vi "NET Control Test.vi"() -> ()   [LabVIEW 2012]
uses:
  NationalInstruments.VeriStand.SystemStorageUI
  NationalInstruments.VeriStand.SystemDefinitionAPI
  NationalInstruments.VeriStand.SystemStorage
  <vilib>/NI VeriStand/UI Controls/Single Node Browser/NI_VS UI Single Node Browser.lvlib
panel:
  out "Numeric":dbl
  in  "Start Trigger Channel":string
  in  "Select Start Trig":bool
  in  "stop":bool
  in  "Path":path=path "C:/Users/Public/Documents/National Instruments/NI VeriStand 2012/Projects/Untitled 1/Untitled 1.nivssdf"
  in  "Source Waveform":refnum<k24>(container)
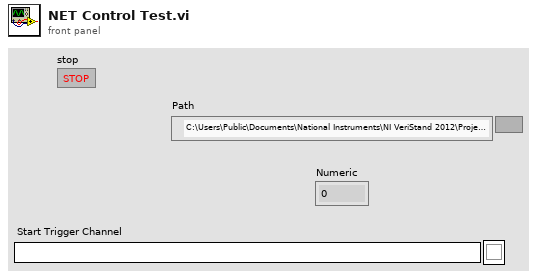
[diagram p1: front panel]
types:
  T1 = typedef "NI_VS UI Single Node Browser.lvlib/Callback Type.ctl" = cluster{"Net Callbacks":refnum<k27>[], "Event":refnum<user-event>}
  T2 = typedef "NI_VS UI Single Node Browser.lvlib/Single Node Browser Ref.ctl" = refnum<k24>
  T3 = typedef "NI_VS UI Single Node Browser.lvlib/Net Event.ctl" = enum16{"SelectedItem"}
  T4 = typedef "NI_VS UI Single Node Browser.lvlib/Node Ref.ctl" = refnum<k24>
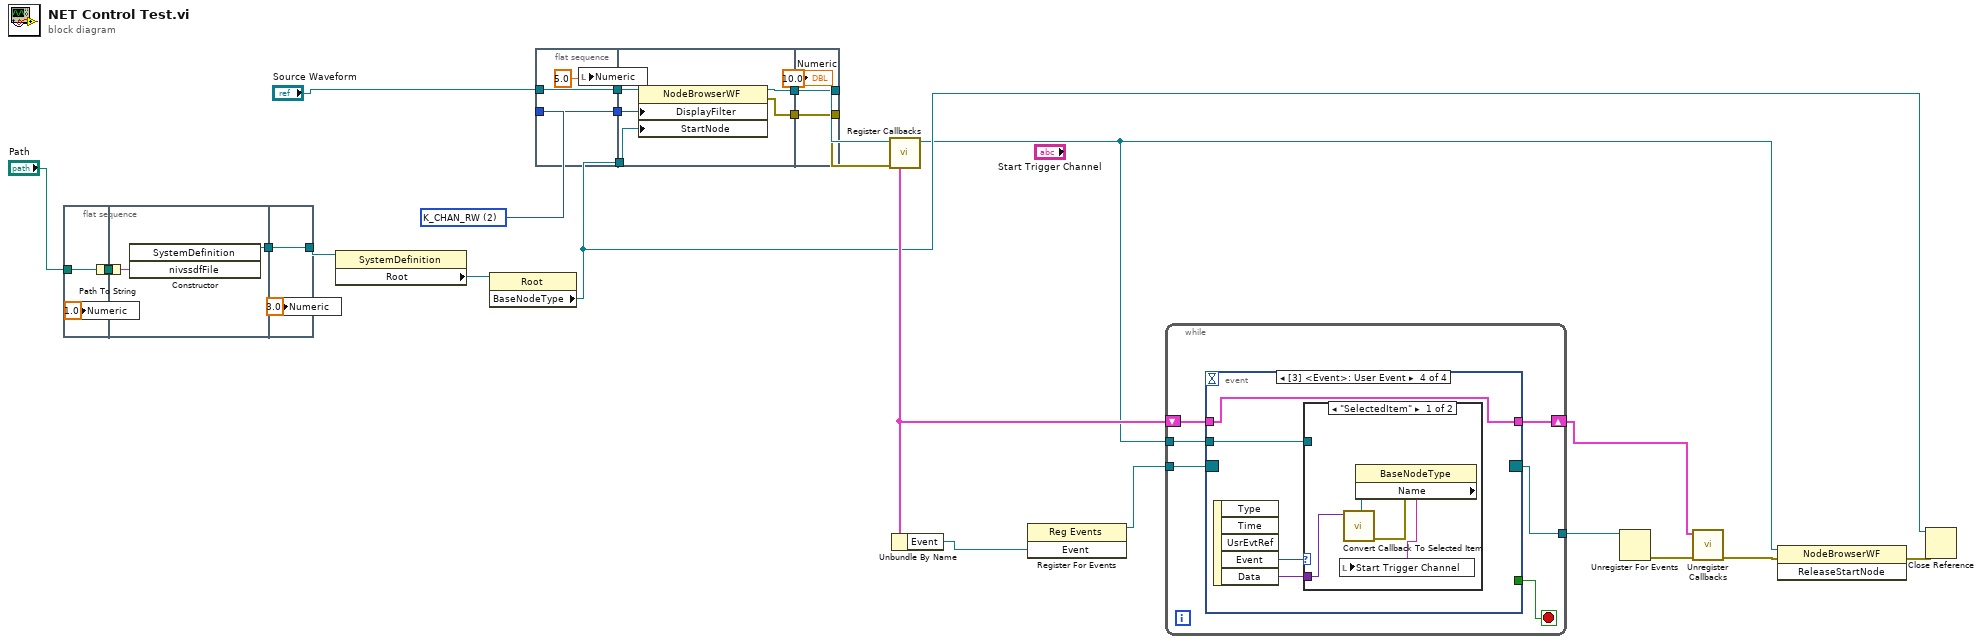
[diagram p0: block diagram]
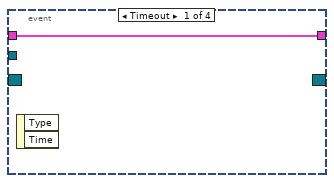
[diagram p2: hidden frame]
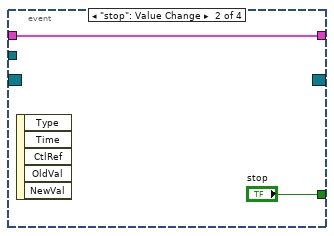
[diagram p3: hidden frame]
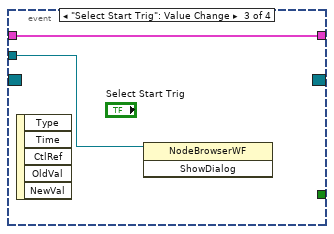
[diagram p4: hidden frame]
diagram:
  w19 = u8 2 items=["K_CHAN_R", "K_CHAN_W", "K_CHAN_RW", "K_CHAN_VOLT", "K_CHAN_FAULT", "K_ALL", "K_CUSTOM", "K_CHAN_R_VIS", "K_CHAN_W_VIS", "K_CHAN_RW_VIS", "K_CHAN_VOLT_VIS", "K_CHAN_FAULT_VIS", "K_WAVE", "K_WAVE_VIS", "K_WAVE_DBL", "K_WAVE_CDB", "K_WAVE_DBL_VIS", "K_WAVE_CDB_VIS"] ("DisplayFilter")
  n1 = flat-sequence {
    tunnel: "Path" -> [w25]
    tunnel: [w25] -> w2
    tunnel: w2 -> [w28]
    tunnel: [w26] -> w1
    tunnel: [w30] -> w21
    tunnel: w1 -> [w30]
    frame #0 {
      n2 = local write "Numeric"(1.0 ("Numeric")) -> ()
    }
    frame #1 {
      n3 = Path To String(path=w28) -> (string=w27:string)
      n4 = constructor class="SystemDefinition"("nivssdfFile"=w27) -> (reference out=w26:refnum<k24>)  [unwired: 3 in, 3 out]
    }
    frame #2 {
      n5 = local write "Numeric"(3.0 ("Numeric")) -> ()
    }
  }
  n6 = property class="SystemDefinition"(reference=w21) -> ("Root"=w20:refnum<k24>)  [unwired: 1 in, 2 out]
  n7 = property class="Root"(reference=w20) -> ("BaseNodeType"=w9:refnum<k24>)  [unwired: 1 in, 2 out]
  n8 = flat-sequence {
    tunnel: w19 -> [w32]
    tunnel: "Source Waveform" -> [w33]
    tunnel: [w33] -> w6
    tunnel: [w32] -> w5
    tunnel: w9 -> [w35]
    tunnel: w6 -> [w38]
    tunnel: w5 -> [w37]
    tunnel: [w36] -> w4
    tunnel: [w34] -> w3
    tunnel: [w40] -> w7
    tunnel: [w41] -> w18
    tunnel: w4 -> [w41]
    tunnel: w3 -> [w40]
    frame #0 {
      n9 = local write "Numeric"(5.0 ("Numeric")) -> ()
    }
    frame #1 {
      n10 = property class="NodeBrowserWF"(reference=w38, "DisplayFilter"=w37, "StartNode"=w35) -> (reference out=w36:refnum<k24>, error out=w34:errorcluster)  [unwired: 1 in]
    }
    frame #2 {
      "Numeric" <- 10.0 ("Numeric")
    }
  }
  n11 = call <vilib>:"Register Callbacks.vi"("error in (no error)"=w7, "Single Node Browser"=w18) -> ("Callbacks"=w14:T1, "Single Node Browser dup"=w8:T2)  [unwired: 7 in, 1 out]
  n12 = Unbundle By Name(w14) -> ("Event"=w17:refnum<user-event>)
  n13 = register-events(w17) -> (reference out=w16:refnum<event-registration>)  [unwired: 2 in, 1 out]
  n14 = while {
    tunnel: w16 -> [w46]
    tunnel: [w45] -> w15
    shift-right: [w44] -> w13
    shift-left: w14 -> [w43]
    tunnel: w8 -> [w42]
    stop <- w47 stop-if-true
    n15 = event shown="[3] <Event>: User Event" {
      selector: w46 -> [_ _ _ _]
      dyn-events: [_ _ _ _] -> w45
      timeout: _ -> [_ _ _ _]
      tunnel: [_ "stop" _ _] -> w47
      tunnel: [w48 w49 w52 w54] -> w44
      tunnel: w43 -> [w48 w49 w52 w54]
      tunnel: w42 -> [_ _ w51 w53]
      event Timeout {
        n16 = event-data() -> ()  [unwired: 1 in, 2 out]
      }
      event "stop": Value Change {
        n17 = event-data() -> ()  [unwired: 1 in, 5 out]
      }
      event "Select Start Trig": Value Change {
        n18 = event-data() -> ()  [unwired: 1 in, 5 out]
        n19 = invoke class="NodeBrowserWF" method="ShowDialog"(reference=w51) -> ()  [unwired: 2 in, 3 out]
      }
      event User Event {
        n20 = event-data() -> ("Event"=w56:T3, "Data"=w55:variant)  [unwired: 1 in, 3 out]
        n21 = case shown="\"SelectedItem\"" w56 {
          tunnel: w55 -> [w60 _]
          tunnel: w53 -> [_ _]
          frame "SelectedItem" {
            n22 = call <vilib>:"Convert Callback To Selected Item.vi"("Data"=w60) -> ("error out"=w59:errorcluster, "Selected Item"=w58:T4)  [unwired: 9 in]
            n23 = property class="BaseNodeType"(reference=w58, error in=w59) -> ("Name"=w57:string)  [unwired: 2 out]
            n24 = local write "Start Trigger Channel"(w57) -> ()
          }
          frame Default {
          }
        }
      }
    }
  }
  n25 = Unregister For Events(event registration refnum=w15) -> (error out=w12:errorcluster)  [unwired: 1 in]
  n26 = call <vilib>:"Unregister Callbacks.vi"("error in (no error)"=w12, "Callback"=w13) -> ("error out"=w11:errorcluster)  [unwired: 9 in]
  n27 = invoke class="NodeBrowserWF" method="ReleaseStartNode"(reference=w8, error in=w11) -> (error out=w10:errorcluster)  [unwired: 1 in, 2 out]
  n28 = Close Reference(reference=w9, error in (no error)=w10) -> ()  [unwired: 1 out]
